vi "EXCEL READ AND WRITE.vi"() -> ()   [LabVIEW 2021]
panel:
  in  "POST":enum16{"", "KEEP OPEN", "CLOSE"}(ring)
  in  "WRITE 1":string
  out "READ 1":string
  in  "CELL 1":string
  in  "FUNCTION":enum16{"", "READ", "WRITE"}(ring)
  in  "Excel._Worksheet":refnum<k7>
  in  "SHEET NUMBER":dbl
  in  "Path":path=path "D:/LABVIEW TRIALS/USER.xlsx"
  in  "Excel._Application":refnum<k7>
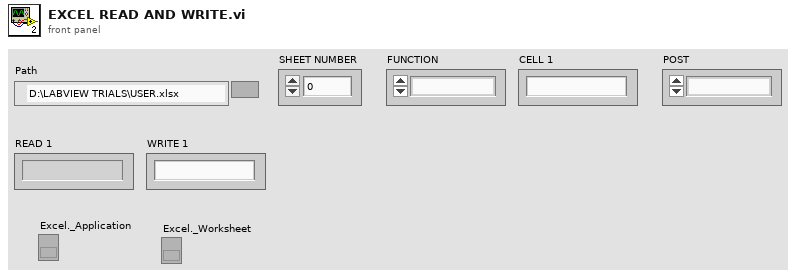
[diagram p1: front panel]
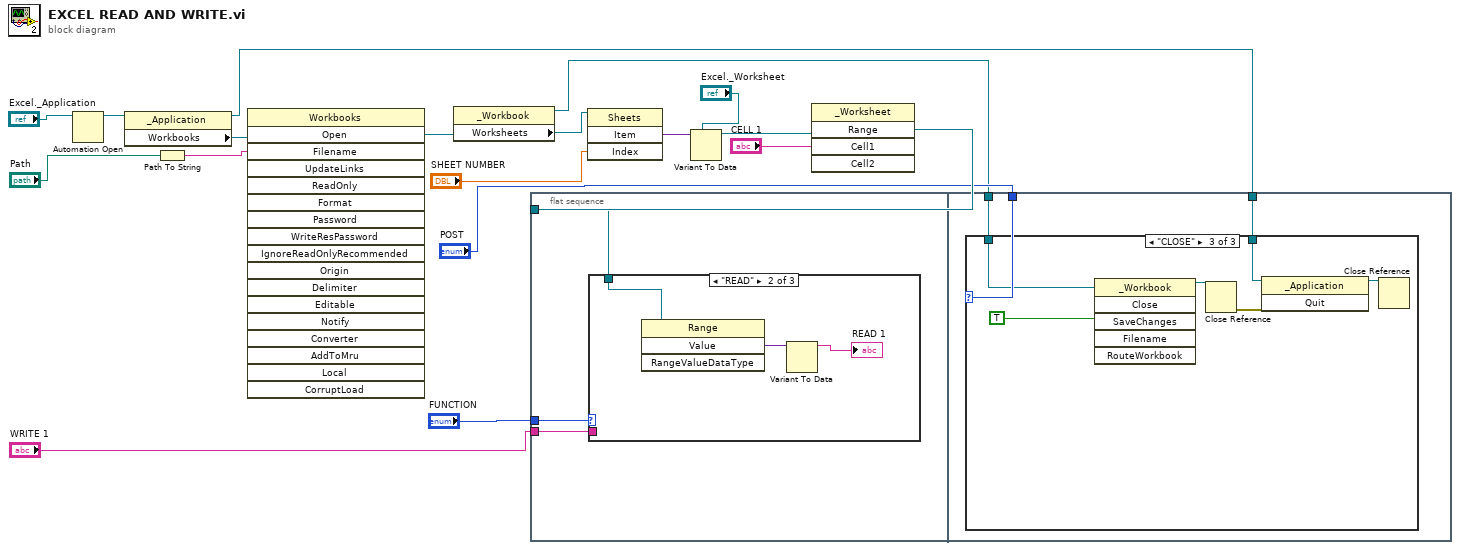
[diagram p0: block diagram]
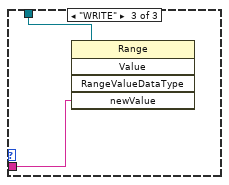
[diagram p3: hidden frame]
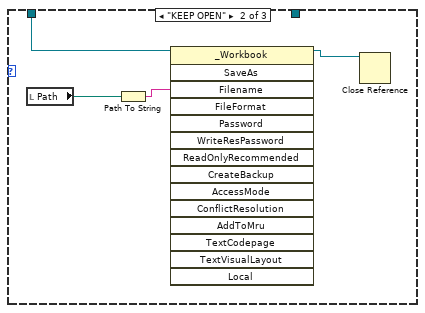
[diagram p5: hidden frame]
diagram:
  n1 = Automation Open(Automation Refnum="Excel._Application") -> (Automation Refnum=w17:refnum<k7>)  [unwired: 3 in, 1 out]
  n2 = property class="_Application"(reference=w17) -> (reference out=w1:refnum<k7>, "Workbooks"=w16:refnum<k7>)  [unwired: 1 in, 1 out]
  n3 = Path To String(path="Path") -> (string=w15:string)
  n4 = invoke class="Workbooks" method="Open"(reference=w16, "Filename"=w15) -> ("Open"=w7:refnum<k7>)  [unwired: 16 in, 17 out]
  n5 = property class="_Workbook"(reference=w7) -> (reference out=w2:refnum<k7>, "Worksheets"=w13:refnum<k7>)  [unwired: 1 in, 1 out]
  n6 = flat-sequence {
    tunnel: "FUNCTION" -> [w21]
    tunnel: w5 -> [w20]
    tunnel: "WRITE 1" -> [w19]
    tunnel: "POST" -> [w29]
    tunnel: w2 -> [w28]
    tunnel: w1 -> [w27]
    frame #0 {
      n7 = case shown="\"READ\"" w21 {
        tunnel: w20 -> [_ w24 w26]
        tunnel: w19 -> [_ _ w25]
        frame "" {
        }
        frame "READ" {
          n8 = invoke class="Range" method="Value"(reference=w24) -> ("Value"=w23:variant)  [unwired: 3 in, 3 out]
          n9 = Variant To Data(Variant=w23) -> (data=→"READ 1":string)  [unwired: 2 in, 1 out]
        }
        frame "WRITE" {
          n10 = invoke class="Range" method="Value"(reference=w26, "newValue"=w25) -> ()  [unwired: 3 in, 5 out]
        }
      }
    }
    frame #1 {
      n11 = case shown="\"CLOSE\"" w29 {
        tunnel: w28 -> [_ w33 w39]
        tunnel: w27 -> [_ _ w35]
        frame "" {
        }
        frame "KEEP OPEN" {
          n12 = local read "Path"() -> (w32:path)
          n13 = Path To String(path=w32) -> (string=w31:string)
          n14 = invoke class="_Workbook" method="SaveAs"(reference=w33, "Filename"=w31) -> (reference out=w30:refnum<k7>)  [unwired: 13 in, 14 out]
          n15 = Close Reference(reference=w30) -> ()  [unwired: 1 in, 1 out]
        }
        frame "CLOSE" {
          n16 = invoke class="_Workbook" method="Close"(reference=w39, "SaveChanges"=TRUE) -> (reference out=w37:refnum<k7>)  [unwired: 4 in, 5 out]
          n17 = Close Reference(reference=w37) -> (error out=w36:errorcluster)  [unwired: 1 in]
          n18 = invoke class="_Application" method="Quit"(reference=w35, error in=w36) -> (reference out=w34:refnum<k7>)  [unwired: 1 in, 2 out]
          n19 = Close Reference(reference=w34) -> ()  [unwired: 1 in, 1 out]
        }
      }
    }
  }
  n20 = invoke class="Sheets" method="Item"(reference=w13, "Index"="SHEET NUMBER") -> ("Item"=w11:variant)  [unwired: 2 in, 3 out]
  n21 = Variant To Data(type="Excel._Worksheet", Variant=w11) -> (data=w9:refnum<k7>)  [unwired: 1 in, 1 out]
  n22 = invoke class="_Worksheet" method="Range"(reference=w9, "Cell1"="CELL 1") -> ("Range"=w5:refnum<k7>)  [unwired: 3 in, 4 out]
